vi "Pic Overlay b Box.vi"(8 "error in (no error)":errorcluster, 10 "Picture in":picture, 11 "LF2R IDE in":refnum<class "Main Panel.lvclass">) -> (0 "error out":errorcluster, 2 "Picture out":picture, 3 "LF2R IDE out":refnum<class "Main Panel.lvclass">)   [LabVIEW 2018, in "Main Panel.lvlib" / "Main Panel.lvclass"]
uses:
  Main Panel.lvclass
  Main Panel.lvclass/Main Panel.ctl
  Picture Process/Picture Process.lvclass
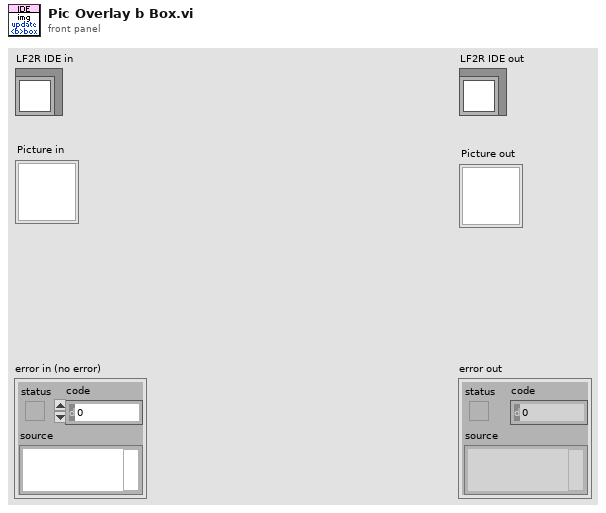
[diagram p1: front panel]
types:
  T1 = typedef "Data Parser.lvclass/frame b data.ctl" = cluster{"kind":string, "x":string, "y":string, "w":string, "h":string}
  T2 = cluster{"Fill Color":u32, "Border Color":u32, "Show?":bool}
  T3 = cluster{"x":string, "y":string, "w":string, "h":string}
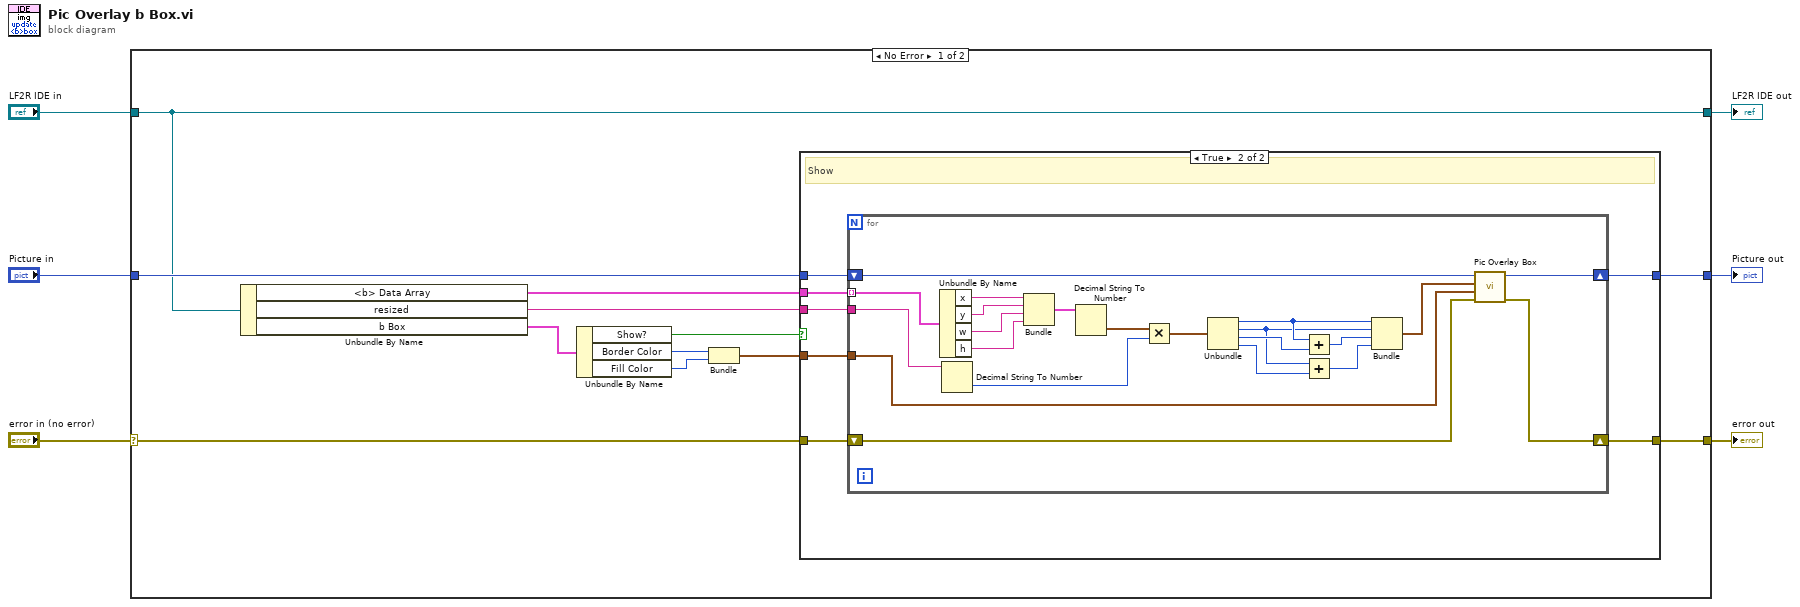
[diagram p0: block diagram]
diagram:
  n1 = case shown="No Error" "error in (no error)" {
    selector: "error in (no error)" -> [w11 w52]
    tunnel: [w8 w52] -> w5
    tunnel: [w7 w51] -> w3
    tunnel: "LF2R IDE in" -> [w7 w51]
    tunnel: "Picture in" -> [w10 w50]
    tunnel: [w9 w50] -> w1
    frame No Error {
      n2 = Unbundle By Name(w7) -> ("<b> Data Array"=w18:T1[], "resized"=w17:string, "b Box"=w16:T2)
      n3 = Unbundle By Name(w16) -> ("Show?"=w15:bool, "Border Color"=w14:u32, "Fill Color"=w13:u32)
      n4 = Bundle("Border Color"=w14, "Fill Color"=w13) -> (w12:cluster{"Border Color":u32, "Fill Color":u32})  [unwired: 1 in]
      n5 = case shown="True" w15 {
        tunnel: w18 -> [_ w27]
        tunnel: w11 -> [w20 w21]
        tunnel: [w20 w22] -> w8
        tunnel: w17 -> [_ w26]
        tunnel: w12 -> [_ w25]
        tunnel: w10 -> [w19 w24]
        tunnel: [w19 w23] -> w9
        frame False {
          # "Skip"
        }
        frame True {
          # "Show"
          n6 = for {
            tunnel: w27 -> [w49] mode=indexing
            shift-right: [w29] -> w22
            shift-left: w21 -> [w30]
            shift-right: [w28] -> w23
            shift-left: w24 -> [w33]
            tunnel: w26 -> [w35]
            tunnel: w25 -> [w31]
            n7 = Unbundle By Name(w49) -> ("x"=w46:string, "y"=w45:string, "w"=w44:string, "h"=w43:string)
            n8 = Decimal String To Number(string=w35) -> (number=w34:i32)  [unwired: 2 in, 1 out]
            n9 = Bundle("x"=w46, "y"=w45, "w"=w44, "h"=w43) -> (w42:T3)  [unwired: 1 in]
            n10 = Decimal String To Number(string=w42) -> (number=w37:cluster{"x":i32, "y":i32, "w":i32, "h":i32})  [unwired: 2 in, 1 out]
            n11 = Multiply(x=w37, y=w34) -> (x*y=w36:cluster{"x":i32, "y":i32, "w":i32, "h":i32})
            n12 = Unbundle(w36) -> ("x"=w41:i32, "y"=w39:i32, "w"=w40:i32, "h"=w38:i32)
            n13 = Add(x=w41, y=w40) -> (x+y=w48:i32)
            n14 = Add(x=w39, y=w38) -> (x+y=w47:i32)
            n15 = Bundle("x"=w41, "y"=w39, w48, w47) -> (w32:cluster{"x":i32, "y":i32, i32, i32})  [unwired: 1 in]
            n16 = call "Pic Overlay Box.vi"("error in (no error)"=w30, "Color"=w31, "Rectangle"=w32, "Picture in"=w33) -> ("error out"=w29:errorcluster, "Picture out"=w28:picture)  [unwired: 6 in]
          }
        }
      }
    }
    frame Error {
    }
  }
  "error out" <- w5
  "LF2R IDE out" <- w3
  "Picture out" <- w1
